vi "ExCenterStripSpecFw.vi"() -> ()   [LabVIEW 2010]
panel:
  in  "Filter":i16=1 min=1 max=100 step=1
  in  "Wavelength":dbl=546.0 format="%.2f"
  in  "Grating Speed":dbl=2000.0 min=1.0 step=1.0 format="%.2f"
  in  "Grating number":i16=1 min=1 max=100 step=1
  out "Strip":sgl[](graph)
  in  "Temperature":dbl=-10.0 format="%.2f"
  in  "Exposure":dbl=0.5 min=0.0 step=0.001 format="%.3f"
  in  "stop":bool
  out "error out":errorcluster
  in  "error in (no error)":errorcluster
  # "ExCenterStripSpecFw.vi\n(Normal Spectrograph and Filter Wheel via 2 different USB/COM ports)\nCamera, Spectrometer and Filter Wheel control.  This vi will open the camera, spectrograph and filter wheel.  It will then move the grating to the Wavelength and set the Filter.  Data will then be collected and displayed until the STOP button is hit."
  # "NOTES:\nA properly configured spectometer .ini must be present in the LabVIEW folder for spectrograph operation.\n\nConsult the Toolkit documentation for more information on how to configure this file."
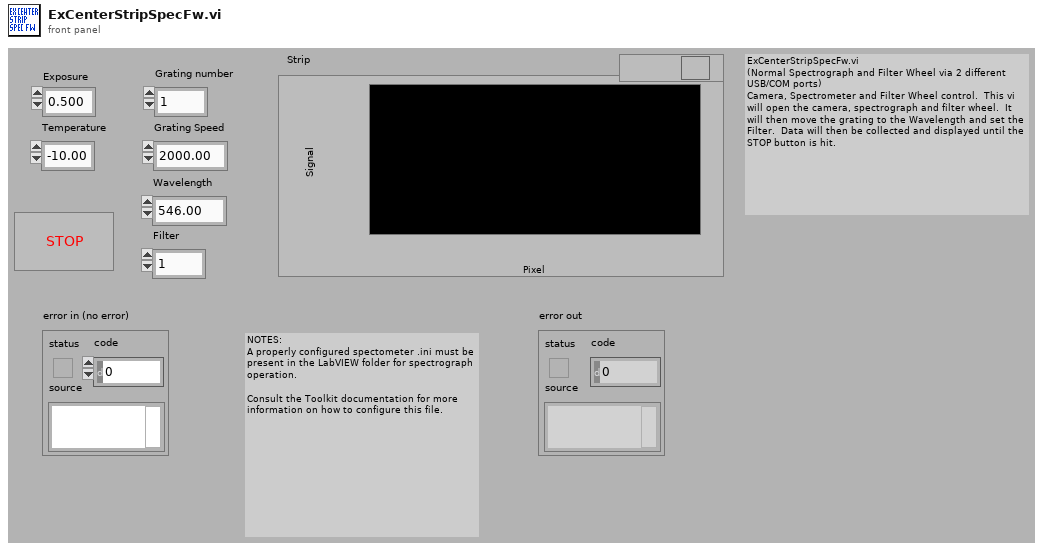
[diagram p1: front panel]
types:
  T1 = cluster{"acquire focus mode":u32, "Exposure":dbl, "Number of Images":u32, "Software accumulation":u32}
  T2 = cluster{"Camera Handle":u32, "Pulser Handle":u32, "File Handle":u32, "Display Handle":u32, "Image Handle":u32}
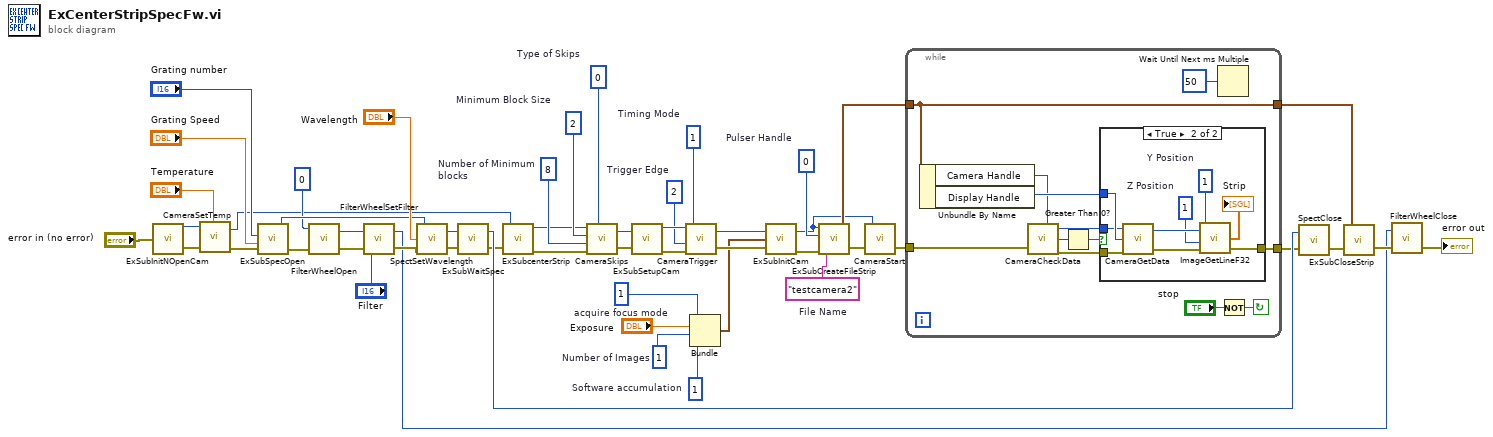
[diagram p0: block diagram]
diagram:
  w22 = u32 0  # Pulser Handle
  w27 = u32 1  # acquire focus mode
  w26 = u32 1  # Number of Images
  w25 = u32 1  # Software accumulation
  w24 = u32 1  # Timing Mode
  w28 = u32 2  # Trigger Edge
  w30 = u32 0  # Type of Skips
  w31 = u32 2  # Minimum Block Size
  w29 = u32 8  # Number of Minimum blocks
  w20 = "testcamera2"  # File Name
  n1 = call "ExSubInitNOpenCam.vi"("error in (no error)"="error in (no error)") -> ("Camera Handle"=w4:u32, "error out"=w3:errorcluster)
  n2 = call <userlib>:"CameraSetTemp.vi"("error in (no error)"=w3, "Temperature"="Temperature", "Camera Handle"=w4) -> ("error out"=w2:errorcluster, "Camera Handle"=w5:u32)
  n3 = call "ExSubSpecOpen.vi"("error in (no error)"=w2, "Grating speed"="Grating Speed", "Grating number"="Grating number") -> ("error out"=w14:errorcluster, "Spectrometer Handle"=w35:u32)  [unwired: 1 in, 1 out]
  n4 = call <userlib>:"FilterWheelOpen.vi"("error in"=w14, "Filter Wheel ID"=0) -> ("error out"=w13:errorcluster, "Filter Wheel Handlle"=w10:u32)  [unwired: 1 in]
  n5 = call <userlib>:"FilterWheelSetFilter.vi"("error in"=w13, "Filter"="Filter", "Filter Wheel Handle"=w10) -> ("error out"=w12:errorcluster, "Filter Wheel Handle"=w6:u32)  [unwired: 1 in]
  n6 = call <userlib>:"SpectSetWavelength.vi"("error in"=w12, "Wavelength"="Wavelength", "Spectrometer Handle"=w35) -> ("error out"=w37:errorcluster, "Spectrumeter Handle"=w36:u32)
  n7 = call "ExSubWaitSpec.vi"("error in (no error)"=w37, "Spectrometer Handle"=w36) -> ("error out"=w19:errorcluster, "Spectrometer handle"=w33:u32)
  n8 = call "ExSubcenterStrip.vi"("error in (no error)"=w19, "Camera Handle"=w5) -> ("error out"=w17:errorcluster, "Camera Handle"=w18:u32)
  n9 = call <userlib>:"CameraSkips.vi"("Camera Handle"=w18, "Minimum Block Size"=w31, "Number of Minimum blocks"=w29, "error in"=w17, "Type of Skips"=w30) -> ("Camera Handle"=w43:u32, "error out"=w42:errorcluster)
  n10 = call "ExSubSetupCam.vi"("error in (no error)"=w42, "Camera Handle"=w43) -> ("error out"=w15:errorcluster, "Camera Handle"=w46:u32)
  n11 = call <userlib>:"CameraTrigger.vi"("error in"=w15, "Trigger Edge"=w28, "Timing Mode"=w24, "Camera Handle"=w46) -> ("error out"=w47:errorcluster, "Camera Handle"=w45:u32)
  n12 = Bundle("acquire focus mode"=w27, "Exposure"="Exposure", "Number of Images"=w26, "Software accumulation"=w25) -> (w23:T1)  [unwired: 1 in]
  n13 = call "ExSubInitCam.vi"("error in (no error)"=w47, "Camera Information"=w23, "Camera Handle"=w45) -> ("error out"=w16:errorcluster, "Camera Handle"=w21:u32)
  n14 = call "ExSubCreateFileStrip.vi"("error in (no error)"=w16, "File and Display Name"=w20, "Pulser Handle"=w22, "Camera Handle"=w21) -> ("error out"=w41:errorcluster, "Handles Out"=w49:T2)
  n15 = call <userlib>:"CameraStart.vi"("error in"=w41, "Camera Handle"=w21) -> ("error out"=w44:errorcluster)  [unwired: 1 out]
  n16 = while {
    tunnel: w49 -> [w60]
    tunnel: w44 -> [w59]
    tunnel: [w57] -> w32
    tunnel: [w60] -> w48
    stop <- w61 continue-if-true
    n17 = Unbundle By Name(w60) -> ("Camera Handle"=w52:u32, "Display Handle"=w56:u32)
    n18 = call <userlib>:"CameraCheckData.vi"("Camera Handle"=w52, "error in"=w59) -> ("Camera Handle"=w53:u32, "Number Of Frames Available"=w54:i32, "error out"=w58:errorcluster)
    n19 = Greater Than 0?(x=w54) -> (x > 0?=w55:bool)
    n20 = case shown="True" w55 {
      tunnel: w58 -> [w64 w72]
      tunnel: [w64 w70] -> w57
      tunnel: w56 -> [_ w68]
      tunnel: w53 -> [_ w67]
      frame False {
      }
      frame True {
        w65 = u32 1  # Z Position
        w66 = u32 1  # Y Position
        n21 = call <userlib>:"CameraGetData.vi"("error in"=w72, "Data Handle"=w68, "Camera Handle"=w67) -> ("error out"=w71:errorcluster, "Data Handle"=w69:u32)  [unwired: 1 out]
        n22 = call <userlib>:"ImageGetLineF32.vi"("error in"=w71, "Z Position"=w65, "Y Position"=w66, "Data Handle"=w69) -> ("error out"=w70:errorcluster, "Array F32"=→"Strip":sgl[])  [unwired: 1 out]
      }
    }
    n23 = Wait Until Next ms Multiple(millisecond multiple=u32 50) -> ()  [unwired: 1 out]
    n24 = Not(x="stop") -> (.not. x?=w61:bool)
  }
  n25 = call <userlib>:"SpectClose.vi"("error in"=w32, "Spectrometer Handle"=w33) -> ("error out"=w34:errorcluster)
  n26 = call "ExSubCloseStrip.vi"("error in (no error)"=w34, "Handles In"=w48) -> ("error out"=w8:errorcluster)
  n27 = call <userlib>:"FilterWheelClose.vi"("error in"=w8, "Filter Wheel Handle"=w6) -> ("error out"=→"error out":errorcluster)
